vi "codecForLocale.vi"(8 "Error In":errorcluster) -> (0 "Error Out":errorcluster, 3 "New QTextCodec":refnum<class "QTextCodec.lvclass">)   [LabVIEW 2014, in "QTextCodec.lvclass"]
doc: "LabVIEW-specific documentation is not yet available. See <b>http://doc.qt.io/qt-5/QTextCodec.html#codecForLocale</b>"
uses:
  QTextCodec.lvclass
  LQCoreEngine/_Internal/LQIdentity Registry Action.ctl
  LQIdentity/LQIdentity.lvclass/LQIdentity.ctl
  LQCoreEngine/LQCoreEngine.lvclass
  LQ Core.lvlib
  LQIdentity/LQIdentity.lvclass
panel:
  # "Copyright (c) 2016 Sze Howe Koh\n\nThis Source Code Form is subject to the terms of the Mozilla Public\nLicense, v. 2.0. If a copy of the MPL was not distributed with this\nfile, You can obtain one at http://mozilla.org/MPL/2.0/."
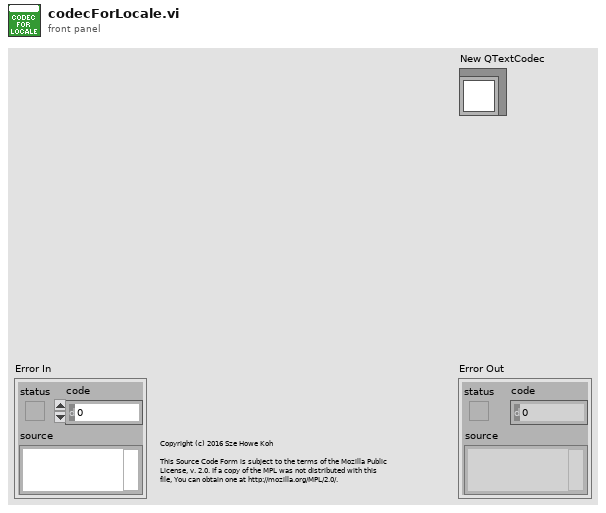
[diagram p1: front panel]
types:
  T1 = typedef "LQ Core.lvlib/LQCoreEngine.lvclass/LQIdentity Registry Action.ctl" = enum16{"Init", "Register LQIdentity", "Get LQIdentity Info", "Deregister LQIdentity"}
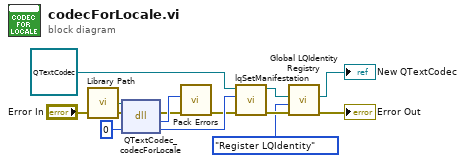
[diagram p0: block diagram]
diagram:
  n1 = call "Library Path.vi"() -> ("Library Path"=w10:path)
  n2 = dll-call lib="?" fn="QTextCodec_codecForLocale"(path in=w10, error in="Error In", "_retVal"=u64 0 ("_instance")) -> (error out=w8:errorcluster, w9:i32, "_retVal"=w11:u64)  [unwired: 1 in, 1 out]
  n3 = call "Pack Errors.vi"("Error In"=w8, "Error Code"=w9) -> ("Error Out"=w7:errorcluster)  [unwired: 9 in]
  n4 = call "lqSetManifestation.vi"("Error In"=w7, "Manifestation"=w11, "LQIdentity in"=refnum<class "QTextCodec.lvclass"> refnum ("QTextCodec")) -> ("Error Out"=w5:errorcluster, "LQIdentity out"=w6:refnum<class "QTextCodec.lvclass">)  [unwired: 7 in]
  n5 = call "Global LQIdentity Registry.vi"("Error In"=w5, "Registry Action"=LQIdentity_Registry_Action."Register LQIdentity", "LQIdentity Info In"=w6) -> ("Error Out"=→"Error Out":errorcluster, "LQIdentity Info Out"=→"New QTextCodec":refnum<class "QTextCodec.lvclass">)  [unwired: 7 in]
